vi "Charger_Action.vi"(6 "error in":errorcluster, 8 "Operation":T2=enum."na", 9 "Charger":T1={"address"="COM13", "position"=0, "setpoint"=7500.0} {"setpoint" min=0.0 max=20000.0 step=100.0; "position" min=0 max=5 step=1}) -> (0 "error out":errorcluster)   [LabVIEW 2020]
uses:
  Battery-Charging-Station/Charger_States_Control.ctl
  Charger_Input Control.ctl
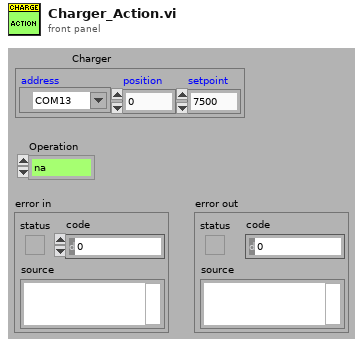
[diagram p1: front panel]
types:
  T1 = typedef "Charger_Input Control.ctl" = cluster{"address":refnum<visa-resource-name>, "position":i32, "setpoint":dbl}
  T2 = typedef "Charger_States_Control.ctl" = enum16{"Enable", "Disable", "Adjust", "Pause", "na"}
  T3 = enum16{"Disable", "Enable", "Update", "Get Info"}
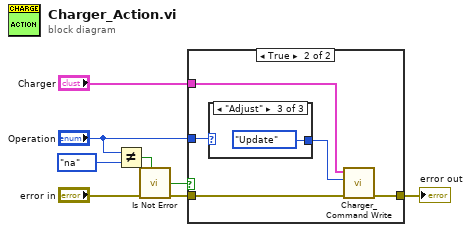
[diagram p0: block diagram]
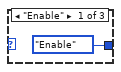
[diagram p3: hidden frame]
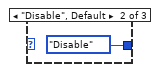
[diagram p4: hidden frame]
diagram:
  n1 = Not Equal?(x="Operation", y=Charger_States_Control."na") -> (x != y?=w4:bool)
  n2 = call "Is Not Error.vi"("enable (T)"=w4, "error in"="error in") -> ("error out"=w6:errorcluster, "ready"=w5:bool)  [unwired: 4 in, 1 out]
  n3 = case shown="True" w5 {
    tunnel: [w9 w14] -> w8
    tunnel: "Operation" -> [_ w13]
    tunnel: w6 -> [w9 w11]
    tunnel: "Charger" -> [_ w10]
    frame False {
    }
    frame True {
      n4 = case shown="\"Adjust\"" w13 {
        tunnel: [T3."Enable" ("Command") T3."Disable" ("Command") T3."Update" ("Command")] -> w12
        frame "Enable" {
        }
        frame "Disable", Default {
        }
        frame "Adjust" {
        }
      }
      n5 = call "Charger_Command Write.vi"("error in"=w11, "Command"=w12, "Charger"=w10) -> ("error out"=w14:errorcluster)  [unwired: 5 in, 1 out]
    }
  }
  "error out" <- w8
